vi "rtp play.vi"(4 "voltage range":dbl, 6 "freq":u32, 7 "rtp stop event ref":refnum<user-event>, 8 "error in (no error)":errorcluster caption="에러 입력(에러 없음)", 10 "waveform data":i8[](array[numeric]), 11 "DW7802 입력":refnum<class "DW7802.lvclass">) -> (0 "error out":errorcluster caption="에러 출력", 3 "DW7802 출력":refnum<class "DW7802.lvclass">)   [LabVIEW 2020, in "DW7802.lvclass"]
uses:
  DW7802.lvclass
  Haptic IC/Haptic IC.lvclass/Haptic IC.ctl
  SubVIs/I2C/Instance VIs/(SubVI)I2C_8Bit-8Bit_Write_Single.vi
  SubVIs/I2C/Instance VIs/(SubVI)I2C_8Bit-8Bit_Read_Single.vi
  Haptic IC/Haptic IC.lvclass
  DW7802.lvclass/DW7802.ctl
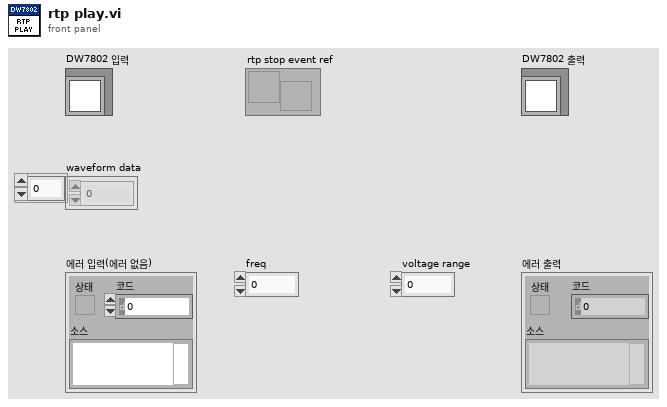
[diagram p1: front panel]
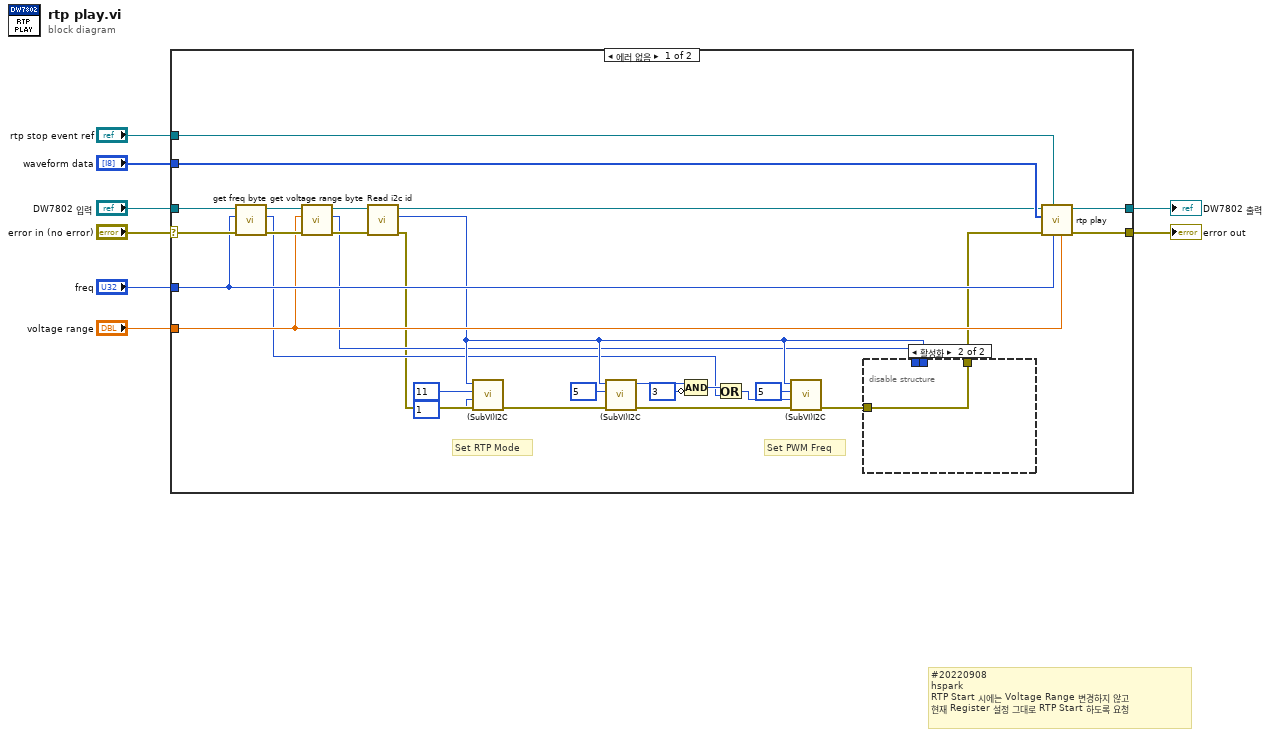
[diagram p0: block diagram]
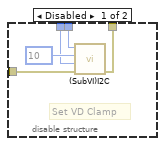
[diagram p2: hidden frame]
diagram:
  # "#20220908\nhspark\nRTP Start 시에는 Voltage Range 변경하지 않고\n현재 Register 설정 그대로 RTP Start 하도록 요청"
  n1 = case shown="에러 없음" "error in (no error)" {
    selector: "error in (no error)" -> [w34 w44]
    tunnel: [w37 w44] -> w8
    tunnel: [w36 w45] -> w7
    tunnel: "voltage range" -> [w28 _]
    tunnel: "freq" -> [w29 _]
    tunnel: "rtp stop event ref" -> [w35 _]
    tunnel: "DW7802 입력" -> [w32 w45]
    tunnel: "waveform data" -> [w33 _]
    frame No Error {
      # "Set PWM Freq"
      # "Set RTP Mode"
      n2 = call-dynamic "get freq byte.vi"("error in (no error)"=w34, "freq"=w29, "DW7802 입력"=w32) -> ("error out"=w31:errorcluster, "byte value"=w12:u8, "DW7802 출력"=w30:refnum<class "DW7802.lvclass">)  [unwired: 6 in]
      n3 = call-dynamic "get voltage range byte.vi"("error in (no error)"=w31, "voltage range"=w28, "DW7802 입력"=w30) -> ("error out"=w27:errorcluster, "byte value"=w11:u8, "DW7802 출력"=w26:refnum<class "DW7802.lvclass">)  [unwired: 6 in]
      n4 = call "Read i2c id.vi"("error in (no error)"=w27, "Haptic IC 입력"=w26) -> ("error out"=w10:errorcluster, "i2c id"=w15:u8, "Haptic IC 출력"=w25:refnum<class "DW7802.lvclass">)  [unwired: 7 in]
      n5 = call-poly "(SubVI)I2C.vi"("error in (no error)"=w10, "Data to Write"=u8 1, "Address"=u8 11, "ID"=w15) -> ("error out"=w18:errorcluster)  [unwired: 6 in, 1 out]
      n6 = call-poly "(SubVI)I2C.vi"("error in (no error)"=w18, "Address"=u8 5, "ID"=w15) -> ("error out"=w22:errorcluster, "Read Data"=w20:u8)  [unwired: 6 in, 1 out]
      n7 = Compound Arithmetic op=AND(w20, invert u8 3 ("y")) -> (w23:u8)
      n8 = Or(x=w23, y=w12) -> (x .or. y?=w13:u8)
      n9 = call-poly "(SubVI)I2C.vi"("error in (no error)"=w22, "Data to Write"=w13, "Address"=u8 5, "ID"=w15) -> ("error out"=w17:errorcluster)  [unwired: 6 in, 1 out]
      n10 = disable-structure shown="활성화" {
        disable-tunnel: w17 -> [w41 w43]
        disable-tunnel: [w40 w43] -> w16
        disable-tunnel: w15 -> [w39 _]
        disable-tunnel: w11 -> [w38 _]
        frame Disabled {
          # "Set VD Clamp"
          n11 = call-poly "(SubVI)I2C.vi"("error in (no error)"=w41, "Data to Write"=w38, "Address"=u8 10, "ID"=w39) -> ("error out"=w40:errorcluster)  [unwired: 6 in, 1 out]
        }
        frame Enabled {
        }
      }
      n12 = call-parent "rtp play.vi"("voltage range"=w28, "freq"=w29, "rtp stop event ref"=w35, "error in (no error)"=w16, "waveform data"=w33, "Haptic IC 입력"=w25) -> ("error out"=w37:errorcluster, "Haptic IC 출력"=w36:refnum<class "DW7802.lvclass">)  [unwired: 4 in]
    }
    frame Error {
    }
  }
  "error out" <- w8
  "DW7802 출력" <- w7
